vi "Counter_Angle_With_Pressure_V1.vi"() -> ()   [LabVIEW 2015]
panel:
  out "Waveform Chart 2":dynamicdata(graph)
  in  "stop":bool
  out "Crank Angle":dbl
  out "Waveform Chart":dbl(graph)
  out "Gauge":dbl(knob) scale=0.0..360.0
  in  "Encoder PPT":dbl
  in  "Encoder Turn Pulse":bool
  out "RPS Value":dbl
  out "time elapsed in Frame 1":u32
  out "millisecond timer value":u32
  in  "stop 2":bool
  out "Boolean 2":bool
  out "Counts":dbl
  in  "Encoder Rising Simulate":bool
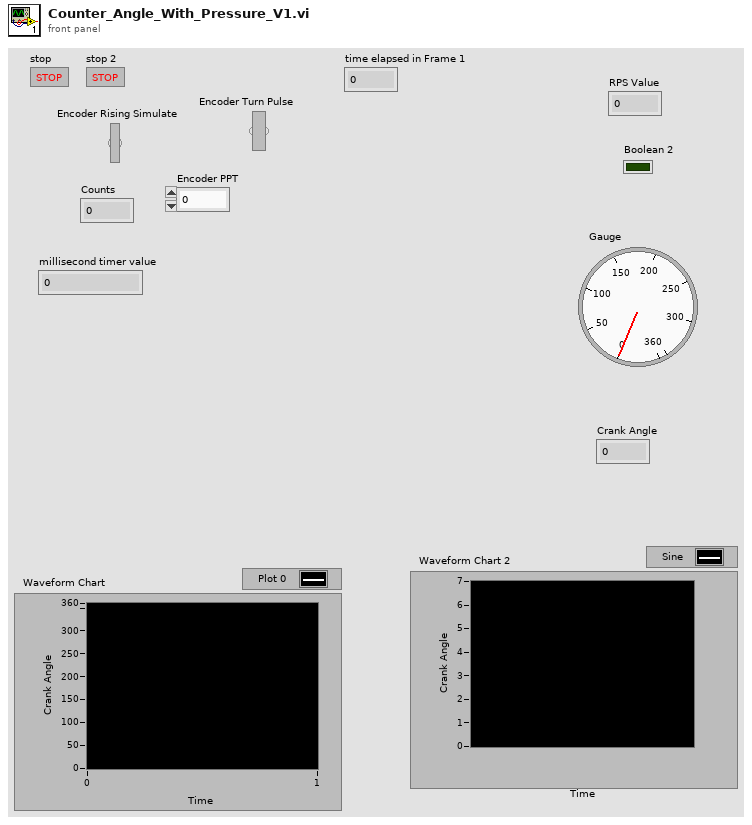
[diagram p1: front panel]
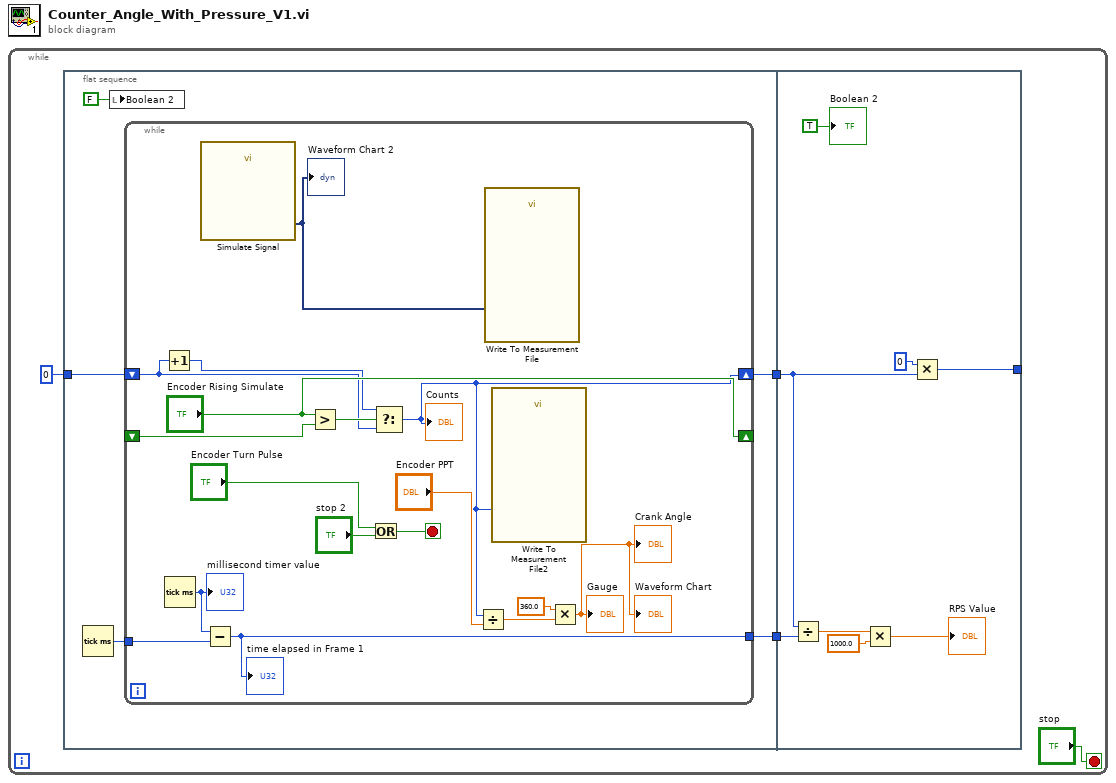
[diagram p0: block diagram]
diagram:
  n1 = while {
    stop <- "stop" stop-if-true
    n2 = flat-sequence {
      tunnel: [w9] -> w4
      tunnel: u8 0 -> [w7]
      tunnel: [w5] -> w2
      tunnel: w4 -> [w27]
      tunnel: w2 -> [w30]
      tunnel: [w29] -> _
      frame #0 {
        n3 = Tick Count (ms)() -> (millisecond timer value=w6:u32)
        n4 = local write "Boolean 2"(FALSE ("Boolean 2")) -> ()
        n5 = while {
          shift-right: ["Encoder Rising Simulate"] -> _
          shift-left: _ -> [w26]
          shift-right: [w10] -> w9
          shift-left: w7 -> [w22]
          tunnel: w6 -> [w20]
          tunnel: [w13] -> w5
          stop <- w12 stop-if-true
          n6 = Increment(x=w22) -> (x+1=w23:u8)
          n7 = Tick Count (ms)() -> (millisecond timer value=w21:u32)
          "millisecond timer value" <- w21
          n8 = call "Simulate Signal"() -> ("Sine"=w11:dynamicdata)  [unwired: 14 in, 1 out]
          "Waveform Chart 2" <- w11
          n9 = Subtract(x=w21, y=w20) -> (x-y=w13:u32)
          "time elapsed in Frame 1" <- w13
          n10 = Greater?(x="Encoder Rising Simulate", y=w26) -> (0:w24:bool)
          n11 = Or(x="Encoder Turn Pulse", y="stop 2") -> (x .or. y?=w12:bool)
          n12 = Select(t=w23, s=w24, f=w22) -> (s? t:f=w10:u8)
          "Counts" <- w10
          n13 = Divide(x=w10, y="Encoder PPT") -> (x/y=w18:dbl)
          n14 = call "Write To Measurement File"("Signals"=w11) -> ()  [unwired: 16 in, 3 out]
          n15 = call "Write To Measurement File2"("Signals"=w10) -> ()  [unwired: 16 in, 3 out]
          n16 = Multiply(x=360.0, y=w18) -> (x*y=→"Gauge" →"Waveform Chart" →"Crank Angle":dbl)
        }
      }
      frame #1 {
        n17 = Divide(x=w27, y=w30) -> (x/y=w32:dbl)
        n18 = Multiply(x=w32, y=1000.0) -> (x*y=→"RPS Value":dbl)
        n19 = Multiply(x=u8 0, y=w27) -> (x*y=w29:u8)
        "Boolean 2" <- TRUE ("Boolean 2")
      }
    }
  }
